vi "Write property metadata.vi"(0 "reference in":refnum<class "TDMS_DataHandler.lvclass">, 5 "error in (no error)":errorcluster) -> (14 "reference out":refnum<class "TDMS_DataHandler.lvclass">, 19 "error out":errorcluster)   [LabVIEW 2019, in "TDMS_DataHandler.lvclass"]
doc: "Write property to channel level metadata"
uses:
  TDMS_DataHandler.lvclass
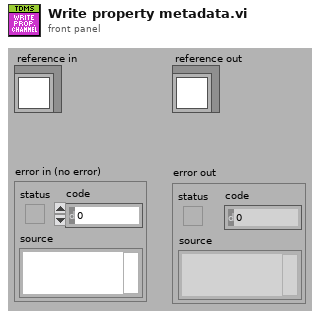
[diagram p1: front panel]
types:
  T1 = typedef "TDMS_DataHandler.lvclass/ObjectAttributes.ctl" = cluster{"Directory":path, "FilePath":path, "FileRef":refnum<k34>, "ExperimentName":string, "GroupName":string, "ChannelNames":string[], "Datum":waveform(dbl)[], "Group_Metadata":cluster{"property names":string[], "property values":variant[]}, "Channel_Metadata":cluster{"property names":string[], "property values":variant[]}}
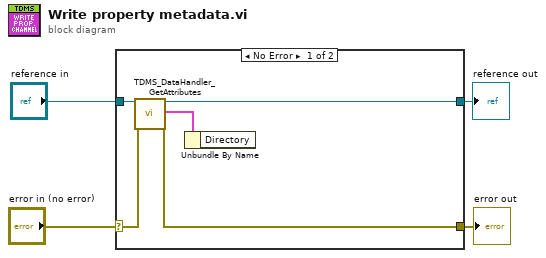
[diagram p0: block diagram]
diagram:
  n1 = case shown="No Error" "error in (no error)" {
    selector: "error in (no error)" -> [w9 w11]
    tunnel: [w8 w11] -> w3
    tunnel: [w7 w10] -> w1
    tunnel: "reference in" -> [w5 w10]
    frame No Error {
      n2 = call "TDMS_DataHandler_GetAttributes.vi"("reference in"=w5, "error in (no error)"=w9) -> ("reference out"=w7:refnum<class "TDMS_DataHandler.lvclass">, "attributes"=w6:T1, "error out"=w8:errorcluster)  [unwired: 14 in, 1 out]
      n3 = Unbundle By Name(w6) -> ()  [unwired: 1 out]
    }
    frame Error {
    }
  }
  "error out" <- w3
  "reference out" <- w1
